vi "Error159.vi"(8 "error in":errorcluster, 11 "Channel":tag) -> (0 "error out":errorcluster, 2 "Channel out":tag)   [LabVIEW 2016]
doc: "Подпрограмма принимает\nи передает на выход список физ. каналов.\nЕсли этот список пустой -\nгенерирует ошибку №159"
panel:
  # "Подпрограмма принимает\nи передает на выход список физ. каналов.\nЕсли этот список пустой -\nгенерирует ошибку №159"
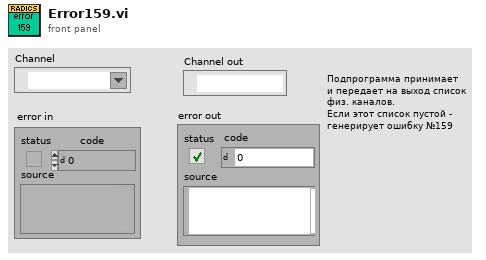
[diagram p1: front panel]
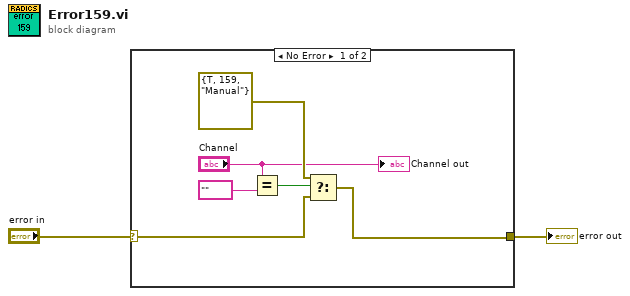
[diagram p0: block diagram]
diagram:
  n1 = case shown="No Error" "error in" {
    selector: "error in" -> [w3 w9]
    tunnel: [w8 w9] -> w2
    frame No Error {
      n2 = Equal?(x="Channel", y=tag "" ("Channels")) -> (x = y?=w6:bool)
      n3 = Select(t=errorcluster {"status"=TRUE, "code"=159, "source"="Manual"} ("error constant"), s=w6, f=w3) -> (s? t:f=w8:errorcluster)
      "Channel out" <- "Channel"
    }
    frame Error {
    }
  }
  "error out" <- w2
